vi "attribute_write_int32.vi"(5 "Repeated Capability":string, 7 "Attribute":T1={"Identifier"="", "Descriptive name"="", "Data Type"=enum."Integer 32", "Command"="", "Access"=2, "Range Table"="", "Read Callback"="", "Write Callback"="", "Range Callback"="", "Check Callback"="", "Rngtable Callback"="", "Coerce Callback"="", "Supported Models"="", "Instrument Options"="", "Repeated Capabilities"="", "Check Status Callback"="", "Index"=0, "Flag: OPC Wait"=FALSE, "Flag: Dont check status"=FALSE, "Flag: Cache Only"=FALSE} {"Access" items=["Read Only", "Write Only", "Read/Write"]}, 8 "error in":errorcluster, 10 "int32 in":i32, 11 "VISA resource name":refnum<visa-resource-name>) -> (0 "error out":errorcluster, 3 "VISA resource name out":refnum<visa-resource-name>)   [LabVIEW 2014, in "rszvl_rsidr_core.lvlib"]
uses:
  rszvl_rsidr_core.lvlib
  type_Attribute.ctl
  type_Attribute_Data_Type.ctl
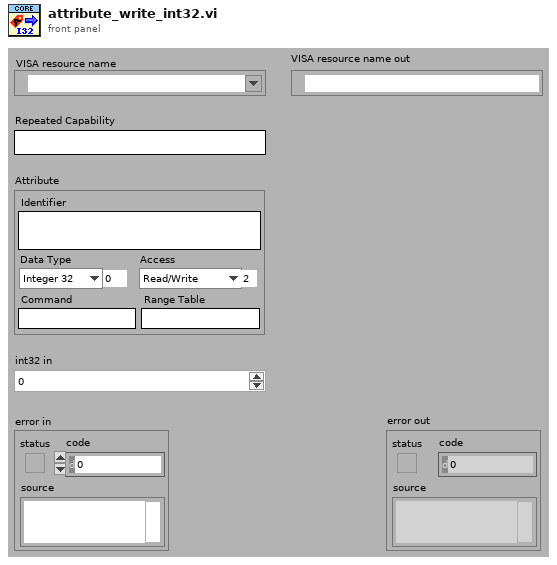
[diagram p1: front panel]
types:
  T1 = typedef "rszvl_rsidr_core.lvlib/type_Attribute.ctl" = cluster{"Identifier":string, "Descriptive name":string, "Data Type":T2, "Command":string, "Access":u16, "Range Table":string, "Read Callback":string, "Write Callback":string, "Range Callback":string, "Check Callback":string, "Rngtable Callback":string, "Coerce Callback":string, "Supported Models":string, "Instrument Options":string, "Repeated Capabilities":string, "Check Status Callback":string, "Index":i32, "Flag: OPC Wait":bool, "Flag: Dont check status":bool, "Flag: Cache Only":bool}
  T2 = typedef "rszvl_rsidr_core.lvlib/type_Attribute_Data_Type.ctl" = enum16{"Integer 32", "Double", "String", "Boolean", "None", "Integer 64"}
  T3 = typedef "rszvl_rsidr_core.lvlib/type_Session_Data.ctl" = cluster{"Instr type":string, "Instr type for err. msg.":string, "Installed Options":string[], "OPC Timeout":i32, "Query Instrument Status":bool, "Check Range":bool, "Check Options":bool, "Add LF to Write":bool, "Simulate":bool, "Logging":bool, "Logging params":variant, "Interface Type":enum16{"Unknown", "GPIB", "VXI", "GPIB_VXI", "ASRL", "PXI", "TCPIP", "USB", "SOCKET"}, "Fast Sweep":i32, "AdditionalFlags":i32, "WaitBeforeWrite":i32, "WaitBeforeRead":i32, "BinDataChunkSize":i64}
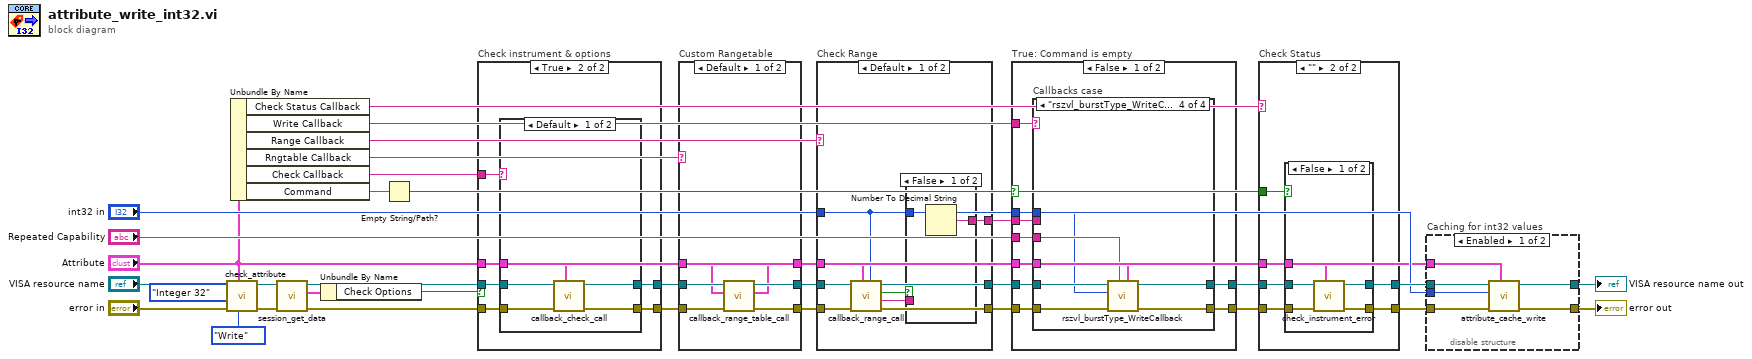
[diagram p0: block diagram]
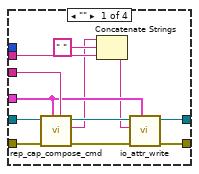
[diagram p2: hidden frame]
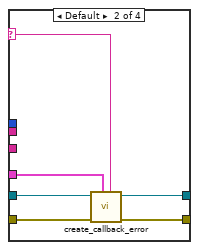
[diagram p3: hidden frame]
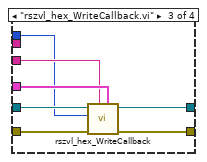
[diagram p4: hidden frame]
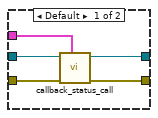
[diagram p6: hidden frame]
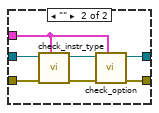
[diagram p9: hidden frame]
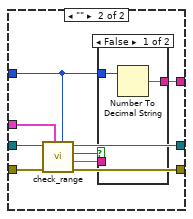
[diagram p12: hidden frame]
diagram:
  n1 = call "check_attribute.vi"("Access"=enum16{"Read", "Write"}."Write", "Attribute"="Attribute", "error in"="error in", "Data Type"=type_Attribute_Data_Type."Integer 32", "VISA resource name"="VISA resource name") -> ("error out"=w10:errorcluster, "VISA resource name out"=w11:refnum<visa-resource-name>)  [unwired: 5 in]
  n2 = Unbundle By Name("Attribute") -> ("Check Status Callback"=w12:string, "Write Callback"=w13:string, "Range Callback"=w15:string, "Rngtable Callback"=w16:string, "Check Callback"=w14:string, "Command"=w1:string)
  n3 = call "session_get_data.vi"("error in"=w10, "VISA resource name"=w11) -> ("error out"=w8:errorcluster, "Session User Data out"=w2:T3, "VISA resource name out"=w9:refnum<visa-resource-name>)  [unwired: 7 in]
  n4 = Unbundle By Name(w2) -> ("Check Options"=w7:bool)
  n5 = Empty String/Path?(string/path=w1) -> (empty?=w31:bool)
  n6 = case "Check instrument & options" shown="True" w7 {
    tunnel: [w36 w42] -> w22
    tunnel: [w35 w41] -> w21
    tunnel: "Attribute" -> [_ w40]
    tunnel: w14 -> [_ w39]
    tunnel: w9 -> [w36 w38]
    tunnel: w8 -> [w35 w37]
    frame False {
    }
    frame True {
      n7 = case shown="Default" w39 {
        tunnel: [w46 w52] -> w42
        tunnel: [w44 w51] -> w41
        tunnel: w37 -> [w45 w50]
        tunnel: w40 -> [w43 w48]
        tunnel: w38 -> [w47 w49]
        frame Default {
          n8 = call "callback_check_call.vi"("Attribute"=w43, "error in"=w45, "VISA resource name"=w47) -> ("error out"=w44:errorcluster, "VISA resource name out"=w46:refnum<visa-resource-name>)  [unwired: 7 in]
        }
        frame "" {
          n9 = call "check_instr_type.vi"("Attribute"=w48, "error in"=w50, "VISA resource name"=w49) -> ("error out"=w54:errorcluster, "VISA resource name out"=w53:refnum<visa-resource-name>)  [unwired: 6 in, 1 out]
          n10 = call "check_option.vi"("Attribute"=w48, "error in"=w54, "VISA resource name"=w53) -> ("error out"=w51:errorcluster, "VISA resource name out"=w52:refnum<visa-resource-name>)  [unwired: 7 in]
        }
      }
    }
  }
  n11 = case "Custom Rangetable" shown="Default" w16 {
    tunnel: w22 -> [w60 w63]
    tunnel: w21 -> [w57 w62]
    tunnel: [w59 w63] -> w20
    tunnel: [w58 w62] -> w19
    tunnel: "Attribute" -> [w56 w61]
    tunnel: [w55 w61] -> w6
    frame Default {
      n12 = call "callback_range_table_call.vi"("error in"=w57, "Attribute in"=w56, "VISA resource name"=w60) -> ("error out"=w58:errorcluster, "Attribute out"=w55:T1, "VISA resource name out"=w59:refnum<visa-resource-name>)  [unwired: 6 in]
    }
    frame "" {
    }
  }
  n13 = case "Check Range" shown="Default" w15 {
    tunnel: w20 -> [w72 w84]
    tunnel: w19 -> [w69 w83]
    tunnel: w6 -> [w65 w77]
    tunnel: [w70 w82] -> w24
    tunnel: [w71 w81] -> w23
    tunnel: "int32 in" -> [w67 w76]
    tunnel: [w66 w78] -> w5
    frame Default {
      n14 = call "callback_range_call.vi"("Attribute Value"=w67, "Attribute"=w65, "error in"=w69, "VISA resource name"=w72) -> ("error out"=w70:errorcluster, "Enum output"=w64:string, "Enum?"=w68:bool, "VISA resource name out"=w71:refnum<visa-resource-name>)  [unwired: 4 in]
      n15 = case shown="False" w68 {
        tunnel: w67 -> [w74 _]
        tunnel: [w73 w75] -> w66
        tunnel: w64 -> [_ w75]
        frame False {
          n16 = Number To Decimal String(number=w74) -> (decimal integer string=w73:string)  [unwired: 1 in]
        }
        frame True {
        }
      }
    }
    frame "" {
      n17 = call "check_range.vi"("Attribute Value"=w76, "Attribute"=w77, "error in"=w83, "VISA resource name"=w84) -> ("error out"=w82:errorcluster, "Enum output"=w79:string, "Enum?"=w80:bool, "VISA resource name out"=w81:refnum<visa-resource-name>)  [unwired: 4 in]
      n18 = case shown="False" w80 {
        tunnel: w76 -> [w86 _]
        tunnel: w79 -> [_ w87]
        tunnel: [w85 w87] -> w78
        frame False {
          n19 = Number To Decimal String(number=w86) -> (decimal integer string=w85:string)  [unwired: 1 in]
        }
        frame True {
        }
      }
    }
  }
  n20 = case "True: Command is empty" shown="False" w31 {
    tunnel: "Repeated Capability" -> [w96 _]
    tunnel: w24 -> [w95 w129]
    tunnel: w23 -> [w94 w130]
    tunnel: "int32 in" -> [w93 _]
    tunnel: w6 -> [w92 _]
    tunnel: w5 -> [w91 _]
    tunnel: [w90 w130] -> w18
    tunnel: [w89 w129] -> w17
    tunnel: w13 -> [w88 _]
    frame False {
      n21 = case "Callbacks case" shown="\"rszvl_burstType_WriteCallback.vi\"" w88 {
        selector: w88 -> [_ w109 _ _]
        tunnel: w93 -> [_ _ w117 w124]
        tunnel: w94 -> [w107 w113 w120 w127]
        tunnel: w95 -> [w105 w114 w121 w128]
        tunnel: w96 -> [w101 _ w118 w125]
        tunnel: [w104 w111 w115 w122] -> w90
        tunnel: [w103 w112 w116 w123] -> w89
        tunnel: w92 -> [w100 w110 w119 w126]
        tunnel: w91 -> [w102 _ _ _]
        frame "" {
          n22 = call "rep_cap_compose_cmd.vi"("Repeated Capability"=w101, "Attribute"=w100, "error in"=w105, "VISA resource name"=w107) -> ("error out"=w106:errorcluster, "Command out"=w97:string, "VISA resource name out"=w108:refnum<visa-resource-name>)  [unwired: 5 in]
          n23 = Concatenate Strings(w97, " ", w102) -> (w98:string)
          n24 = call "io_attr_write.vi"("Attribute"=w100, "error in"=w106, "write buffer"=w98, "VISA resource name"=w108) -> ("error out"=w103:errorcluster, "VISA resource name out"=w104:refnum<visa-resource-name>)  [unwired: 6 in]
        }
        frame Default {
          n25 = call "create_callback_error.vi"("Callback Name"=w109, "Attribute"=w110, "error in"=w114, "VISA resource name"=w113) -> ("error out"=w112:errorcluster, "VISA resource name out"=w111:refnum<visa-resource-name>)  [unwired: 6 in]
        }
        frame "rszvl_hex_WriteCallback.vi" {
          n26 = call "rszvl_hex_WriteCallback.vi"("Attribute"=w119, "Repeated Capability"=w118, "error in"=w121, "Attribute Value I32"=w117, "VISA resource name"=w120) -> ("error out"=w116:errorcluster, "VISA resource name out"=w115:refnum<visa-resource-name>)  [unwired: 5 in]
        }
        frame "rszvl_burstType_WriteCallback.vi" {
          n27 = call "rszvl_burstType_WriteCallback.vi"("Attribute"=w126, "Repeated Capability"=w125, "error in"=w128, "Attribute Value I32"=w124, "VISA resource name"=w127) -> ("error out"=w123:errorcluster, "VISA resource name out"=w122:refnum<visa-resource-name>)  [unwired: 5 in]
        }
      }
    }
    frame True {
    }
  }
  n28 = case "Check Status" shown="\"\"" w12 {
    tunnel: w17 -> [w135 w140]
    tunnel: [w134 w139] -> w30
    tunnel: [w133 w138] -> w29
    tunnel: w18 -> [w132 w141]
    tunnel: w6 -> [w131 w137]
    tunnel: w31 -> [_ w136]
    frame Default {
      n29 = call "callback_status_call.vi"("Attribute"=w131, "error in"=w135, "VISA resource name"=w132) -> ("error out"=w134:errorcluster, "VISA resource name out"=w133:refnum<visa-resource-name>)  [unwired: 7 in]
    }
    frame "" {
      n30 = case shown="False" w136 {
        tunnel: w141 -> [w146 w148]
        tunnel: w140 -> [w145 w147]
        tunnel: [w144 w147] -> w139
        tunnel: [w143 w148] -> w138
        tunnel: w137 -> [w142 _]
        frame False {
          n31 = call "check_instrument_error.vi"("Attribute"=w142, "error in"=w145, "VISA resource name"=w146) -> ("error out"=w144:errorcluster, "VISA resource name out"=w143:refnum<visa-resource-name>)  [unwired: 7 in]
        }
        frame True {
        }
      }
    }
  }
  n32 = disable-structure "Caching for int32 values" shown="Enabled" {
    disable-tunnel: [w154 w156] -> w28
    disable-tunnel: [w153 w155] -> w27
    disable-tunnel: w30 -> [w152 w155]
    disable-tunnel: w29 -> [w151 w156]
    disable-tunnel: "int32 in" -> [w150 _]
    disable-tunnel: "Attribute" -> [w149 _]
    frame Enabled {
      n33 = call "attribute_cache_write.vi"("Attribute"=w149, "error in"=w152, "Value in"=w150, "VISA resource name"=w151) -> ("error out"=w153:errorcluster, "VISA resource name out"=w154:refnum<visa-resource-name>)  [unwired: 6 in]
    }
    frame Disabled {
    }
  }
  "error out" <- w27
  "VISA resource name out" <- w28
